vi "Destroy Win Msg Q.vi"(4 "error in (no error)":errorcluster, 7 "win msg queue":T1) -> (0 "error out":errorcluster)   [LabVIEW 2011]
doc: "Destroys and disposes of a windows message queue. This VI must be called before exiting a VI in which a windows message queue is used.\n\nParameters:\nwin msg queue: the queue to destroy.\n\nErrors:\nReturns 6751 if the queue is not a valid windows message queue."
uses:
  Win Msg Q RefNum.ctl
  lvwinmsg.dll
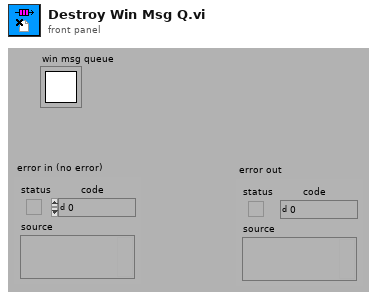
[diagram p1: front panel]
types:
  T1 = typedef "Win Msg Q RefNum.ctl" = refnum<k1>
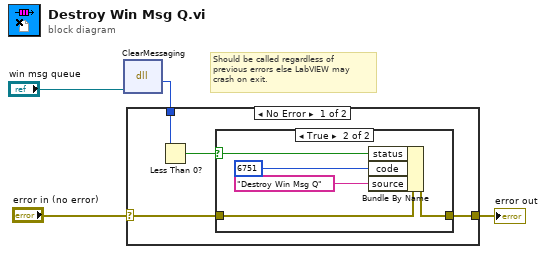
[diagram p0: block diagram]
diagram:
  # "Should be called regardless of\nprevious errors else LabVIEW may\ncrash on exit."
  n1 = dll-call lib="C:/Development/SI.LIB/WIN32/WinMSGQ/lvwinmsg.dll" fn="ClearMessaging"("win msg queue"="win msg queue") -> (w2:i32)  [unwired: 4 in, 2 out]
  n2 = case shown="No Error" "error in (no error)" {
    selector: "error in (no error)" -> [w5 w15]
    tunnel: [w7 w15] -> w4
    tunnel: w2 -> [w6 _]
    frame No Error {
      n3 = Less Than 0?(x=w6) -> (x < 0?=w8:bool)
      n4 = case shown="True" w8 {
        selector: w8 -> [_ w13]
        tunnel: w5 -> [w9 w14]
        tunnel: [w9 w12] -> w7
        frame False {
        }
        frame True {
          n5 = Bundle By Name(cluster=w14, "status"=w13, "code"=6751 ("Error Code"), "source"="Destroy Win Msg Q") -> (w12:errorcluster)
        }
      }
    }
    frame Error {
    }
  }
  "error out" <- w4
